vi "Job Monitor.vi"() -> ()   [LabVIEW 2015]
panel:
  in  "Status":refnum<queue>
  out "UUT_SN":string
  out "Job Folder":path
  in  "Command":refnum<queue>
  in  "Done Button":bool
  out "Status":string[](array[string])
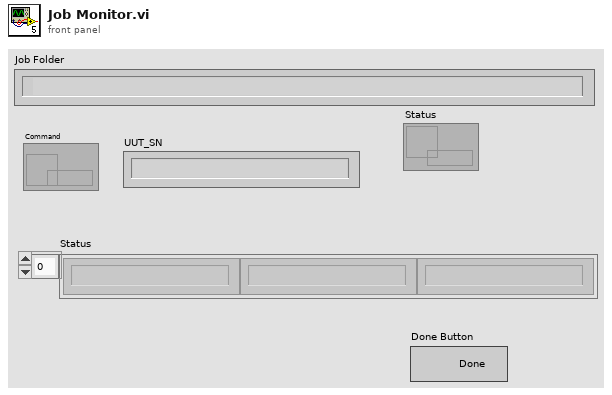
[diagram p1: front panel]
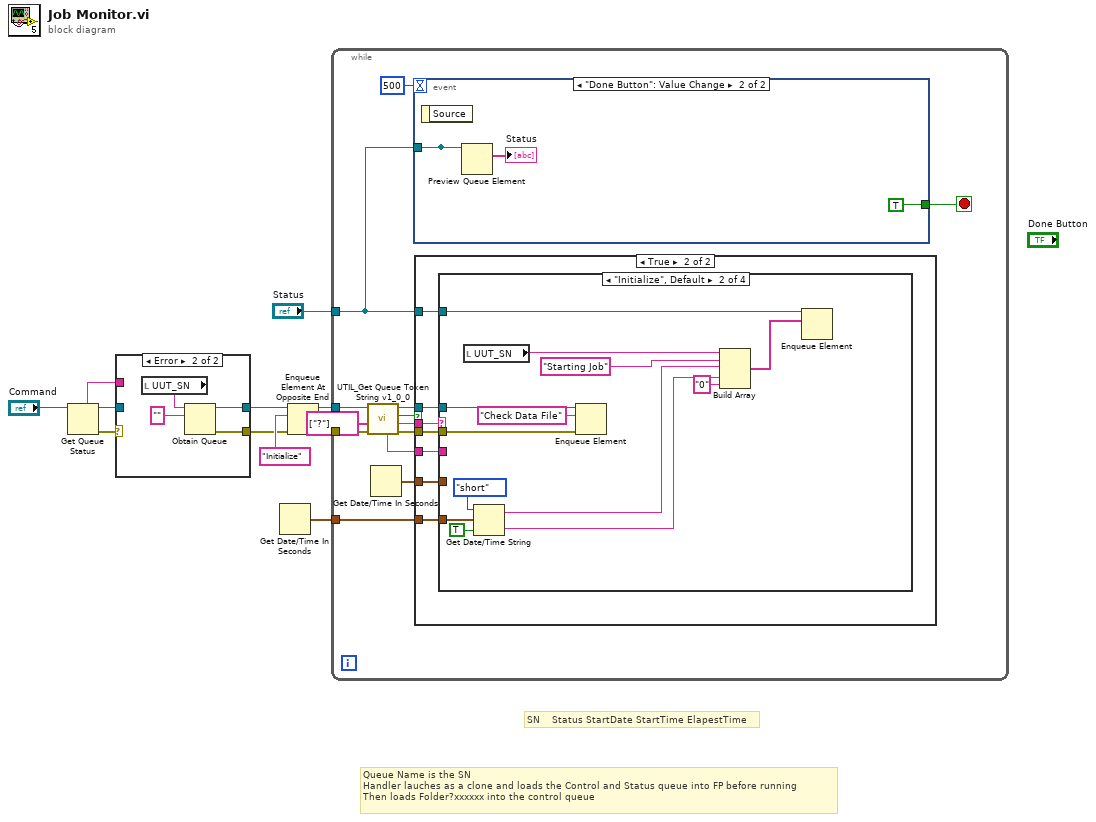
[diagram p0: block diagram]
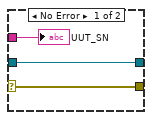
[diagram p2: hidden frame]
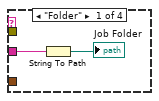
[diagram p4: hidden frame]
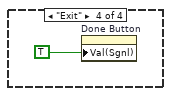
[diagram p6: hidden frame]
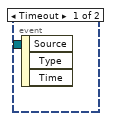
[diagram p7: hidden frame]
diagram:
  # "Queue Name is the SN\nHandler lauches as a clone and loads the Control and Status queue into FP before running\nThen loads Folder?xxxxxx into the control queue"
  # "SN    Status StartDate StartTime ElapestTime"
  n1 = Get Queue Status(queue="Command") -> (queue out=w3:refnum<queue>, queue name=w4:string, error out=w5:errorcluster)  [unwired: 2 in, 5 out]
  n2 = case shown="Error" w5 {
    selector: w5 -> [w13 _]
    tunnel: w4 -> [w14 _]
    tunnel: w3 -> [w12 _]
    tunnel: [w13 w18] -> w2
    tunnel: [w12 w17] -> w1
    frame No Error {
      "UUT_SN" <- w14
    }
    frame Error {
      n3 = local read "UUT_SN"() -> (w15:string)
      n4 = Obtain Queue(name (unnamed)=w15, element data type="") -> (queue out=w17:refnum<queue>, error out=w18:errorcluster)  [unwired: 3 in, 1 out]
    }
  }
  n5 = Get Date/Time In Seconds() -> (seconds since 1Jan1904=w8:timestamp)
  n6 = Enqueue Element At Opposite End(queue=w1, element="Initialize", error in (no error)=w2) -> (queue out=w11:refnum<queue>, error out=w10:errorcluster)  [unwired: 1 in, 1 out]
  n7 = while {
    tunnel: w11 -> [w27]
    tunnel: "Status" -> [w19]
    tunnel: w10 -> [w25]
    tunnel: w8 -> [w23]
    stop <- w30 stop-if-true
    n8 = call "UTIL_Get Queue Token String v1_0_0.vi"("error in (no error)"=w25, "Token"=string[] ["?"], "queue"=w27) -> ("error out"=w24:errorcluster, "token string"=w26:string, "timed out?"=w29:bool, "queue out"=w28:refnum<queue>, "dup string"=w20:string)  [unwired: 1 in, 3 out]
    n9 = Get Date/Time In Seconds() -> (seconds since 1Jan1904=w22:timestamp)
    n10 = event shown="[1] \"Done Button\": Value Change" {
      selector: _ -> [_ _]
      dyn-events: _ -> [_ _]
      timeout: 500 -> [_ _]
      tunnel: [_ TRUE] -> w30
      tunnel: [_ w56] -> _
      tunnel: w19 -> [_ w56]
      event Timeout {
        n11 = event-data() -> ()  [unwired: 1 in, 3 out]
      }
      event "Done Button": Value Change {
        n12 = event-data() -> ()  [unwired: 1 in, 1 out]
        n13 = Preview Queue Element(queue=w56) -> (element=→"Status":string[])  [unwired: 2 in, 3 out]
      }
    }
    n14 = case shown="True" w29 {
      tunnel: w28 -> [_ w36]
      tunnel: w26 -> [_ w38]
      tunnel: w19 -> [_ w37]
      tunnel: w24 -> [_ w35]
      tunnel: w23 -> [_ w34]
      tunnel: w22 -> [_ w33]
      tunnel: w20 -> [_ w32]
      frame False {
      }
      frame True {
        n15 = case shown="\"Initialize\", Default" w38 {
          tunnel: w37 -> [_ w53 _ _]
          tunnel: w36 -> [_ w41 _ _]
          tunnel: w35 -> [_ w42 _ _]
          tunnel: w34 -> [_ w51 _ _]
          tunnel: w33 -> [_ _ _ _]
          tunnel: w32 -> [w40 _ _ _]
          frame "Folder" {
            n16 = String To Path(string=w40) -> (path=→"Job Folder":path)
          }
          frame "Initialize", Default {
            n17 = local read "UUT_SN"() -> (w43:string)
            n18 = Get Date/Time String(date format (0)=enum16{"short", "long", "abbreviated"}."short", seconds (now)=w51, want seconds? (F)=TRUE) -> (date string=w48:string, time string=w47:string)
            n19 = Enqueue Element(queue=w41, element="Check Data File", error in (no error)=w42) -> ()  [unwired: 1 in, 3 out]
            n20 = Build Array(w43, "Starting Job" ("element"), w48, w47, "0" ("element")) -> (w45:string[])
            n21 = Enqueue Element(queue=w53, element=w45) -> ()  [unwired: 2 in, 3 out]
          }
          frame "Check Data File" {
          }
          frame "Exit" {
            n22 = property on="Done Button" class="Bool"("Val(Sgnl)"=TRUE) -> ()  [unwired: 2 in, 2 out]
          }
        }
      }
    }
  }
